vi "WriteCompressed_QDC.vi"(5 "Module":string="data", 7 "name":string, 8 "error in":errorcluster, 10 "Decoded Data":T1[](array[typedef]), 11 "File Handle":T2 format="%.0x") -> (0 "error out":errorcluster)   [LabVIEW 2014]
uses:
  <vilib>/addons/h5labview2/base/hid_t.ctl
  QDCDataCluster.ctl
  <vilib>/addons/h5labview2/base/lib_path.vi
  <vilib>/addons/h5labview2/base/H5Equery.vi
  <vilib>/addons/h5labview2/dataset/H5Dwrite.llb/H5Dwrite.xnode
  <vilib>/addons/h5labview2/space/H5S.lvlib
  <vilib>/addons/h5labview2/dataset/H5D.lvlib
  <vilib>/addons/h5labview2/type/H5T.lvlib
  <vilib>/addons/h5labview2/props/H5P.lvlib
  <vilib>/addons/h5labview2/group/H5G.lvlib
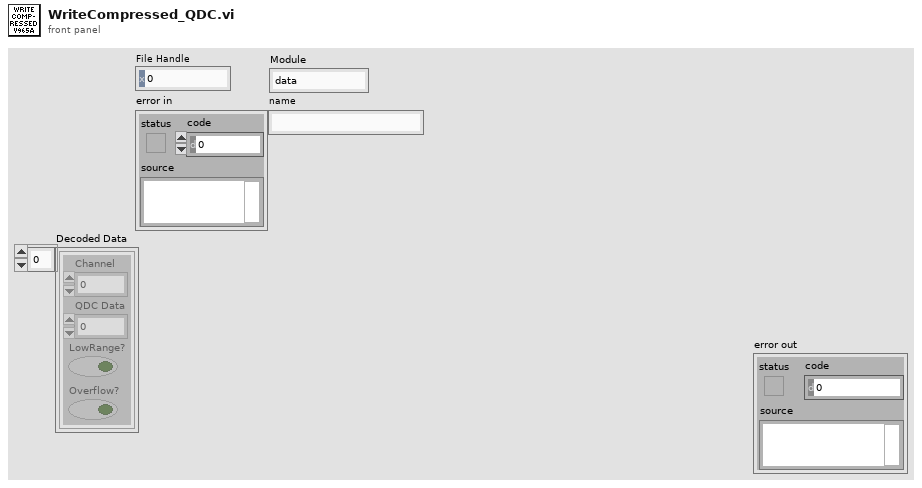
[diagram p1: front panel]
types:
  T1 = typedef "QDCDataCluster.ctl" = cluster{"Channel":u8, "QDC Data":sgl, "LowRange?":bool, "Overflow?":bool}
  T2 = typedef "hid_t.ctl" = i32
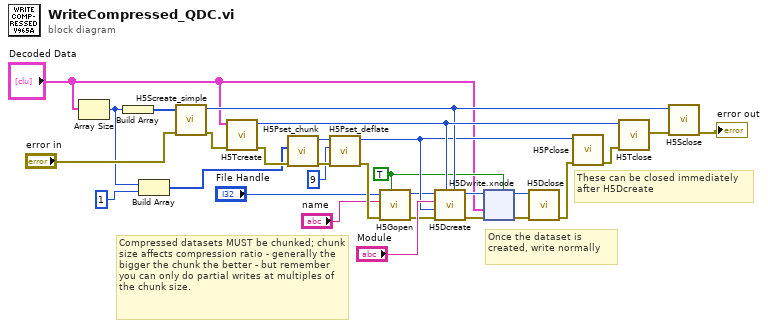
[diagram p0: block diagram]
diagram:
  w7 = TRUE ("create? (F)")
  # "Once the dataset is created, write normally"
  # "Compressed datasets MUST be chunked; chunk size affects compression ratio - generally the bigger the chunk the better - but remember you can only do partial writes at multiples of the chunk size."
  # "These can be closed immediately after H5Dcreate"
  n1 = Array Size(array="Decoded Data") -> (size(s)=w2:i32)
  n2 = Build Array(w2) -> (w4:i32[])
  n3 = Build Array(w2, 1) -> (w1:i32[])
  n4 = call <vilib>:"H5Screate_simple.vi"("error in (no error)"="error in", "dims"=w4) -> ("error out"=w29:errorcluster, "space out"=w22:T2)  [unwired: 7 in, 1 out]
  n5 = call <vilib>:"H5Tcreate.vi"("error in (no error)"=w29, "type variant"="Decoded Data") -> ("error out"=w17:errorcluster, "type out"=w23:i32)  [unwired: 7 in, 1 out]
  n6 = call <vilib>:"H5Pset_chunk.vi"("error in (no error)"=w17, "chunk size"=w1) -> ("error out"=w16:errorcluster, "prop out"=w15:T2)  [unwired: 8 in]
  n7 = call <vilib>:"H5Pset_deflate.vi"("error in (no error)"=w16, "level"=u8 9, "prop in"=w15) -> ("error out"=w11:errorcluster, "prop out"=w19:T2)  [unwired: 7 in]
  n8 = call <vilib>:"H5Gopen.vi"("create? (F)"=w7, "error in (no error)"=w11, "name"="name", "ref in"="File Handle") -> ("error out"=w10:errorcluster, "group out"=w6:T2)  [unwired: 6 in]
  n9 = call <vilib>:"H5Dcreate.vi"("space id"=w22, "type id"=w23, "error in (no error)"=w10, "props id"=w19, "name"="Module", "loc in"=w6) -> ("error out"=w27:errorcluster, "dset out"=w26:T2)  [unwired: 2 in]
  n10 = xnode "H5Dwrite.xnode"("replace? (F)"=w7, "error in (no error)"=w27, "data"="Decoded Data", "ref in"=w26) -> ("error out"=w25:errorcluster, "ref out"=w24:T2)  [unwired: 3 in, 1 out]
  n11 = call <vilib>:"H5Dclose.vi"("error in (no error)"=w25, "dset in"=w24) -> ("error out"=w12:errorcluster)  [unwired: 9 in]
  n12 = call <vilib>:"H5Pclose.vi"("error in (no error)"=w12, "props in"=w19) -> ("error out"=w20:errorcluster)  [unwired: 9 in]
  n13 = call <vilib>:"H5Tclose.vi"("error in (no error)"=w20, "type in"=w23) -> ("error out"=w21:errorcluster)  [unwired: 9 in]
  n14 = call <vilib>:"H5Sclose.vi"("error in (no error)"=w21, "space in"=w22) -> ("error out"=→"error out":errorcluster)  [unwired: 9 in]
